vi "AutoAlign_N664_V2.vi"() -> ()   [LabVIEW 2014]
uses:
  Controls/StageStates.ctl
  Controls/GraphNotifier2D.ctl
panel:
  out "Current Step":i32
  in  "Done":bool
  in  "Repeat":bool
  in  "Start":bool
  out "Cursor Position":dbl=14.501547540983607
  in  "InitialStep":dbl=-0.5
  in  "StepSize":dbl=0.03
  in  "Number Of Steps":i32=35
  out "Intensity Graph":sgl[][](graph)=[[1575.0, 1530.0, 1467.0, 1650.0, 1682.0, 1613.0, 1536.0, 1626.0, 1940.0, 1831.0, 1587.0, 1388.0, 1511.0, 1435.0, 1379.0], [1709.0, 1679.0, 1771.0, 1769.0, 1775.0, 2008.0, 1804.0, 1975.0, 1770.0, 1847.0, 1595.0, 1554.0, 1478.0, 1427.0, 1513.0], [1648.0, 1736.0, 1646.0, 1749.0, 2076.0, 2140.0, 2064.0, 2285.0, 2553.0, 2003.0, 1778.0, 1592.0, 1374.0, 1409.0, 1484.0], [1691.0, 1662.0, 1787.0, 2129.0, 1967.0, 2135.0, 2802.0, 2654.0, 2620.0, 2152.0, 1653.0, 1625.0, 1294.0, 1626.0, 1484.0], [1791.0, 1866.0, 1955.0, 1940.0, 3130.0, 6076.0, 7812.0, 6999.0, 4445.0, 2270.0, 2108.0, 1656.0, 1663.0, 1432.0, 1434.0], [1685.0, 1692.0, 2032.0, 2360.0, 5595.0, 13786.0, 21952.0, 19970.0, 9456.0, 3969.0, 1980.0, 1953.0, 1670.0, 1777.0, 1482.0], [1690.0, 1883.0, 2231.0, 2992.0, 7277.0, 21162.0, 37225.0, 33877.0, 17031.0, 5558.0, 2486.0, 1757.0, 1705.0, 1721.0, 1629.0], [1950.0, 2070.0, 2444.0, 3114.0, 7300.0, 21633.0, 35295.0, 34230.0, 18542.0, 5857.0, 2447.0, 2046.0, 1718.0, 1496.0, 1497.0], [1738.0, 1911.0, 2271.0, 3013.0, 4517.0, 11402.0, 20736.0, 20231.0, 11390.0, 4490.0, 2670.0, 2143.0, 1981.0, 1468.0, 1542.0], [1875.0, 1741.0, 2051.0, 2522.0, 2677.0, 4632.0, 7218.0, 8580.0, 5418.0, 3381.0, 2550.0, 2068.0, 1621.0, 1690.0, 1591.0], [1727.0, 1602.0, 1790.0, 2337.0, 2453.0, 2325.0, 3198.0, 3570.0, 2998.0, 2777.0, 2034.0, 1844.0, 1659.0, 1637.0, 1530.0], [1562.0, 1616.0, 1920.0, 2051.0, 2025.0, 2333.0, 2346.0, 2577.0, 2301.0, 1999.0, 1878.0, 1700.0, 1628.0, 1624.0, 1486.0], [1599.0, 1666.0, 1677.0, 1735.0, 1646.0, 1710.0, 1950.0, 2008.0, 1755.0, 1922.0, 1644.0, 1723.0, 1616.0, 1341.0, 1659.0], [1496.0, 1555.0, 1749.0, 1781.0, 1666.0, 1880.0, 1703.0, 1865.0, 1750.0, 1712.0, 1685.0, 1646.0, 1592.0, 1380.0, 1439.0], [1706.0, 1543.0, 1659.0, 1490.0, 1552.0, 1610.0, 1653.0, 1799.0, 1670.0, 1665.0, 1578.0, 1393.0, 1625.0, 1681.0, 1501.0]]
  in  "Quit":bool
  out "Sample":cluster{dbl[], dbl[]}[](graph)
  in  "Accumulations":i32=10
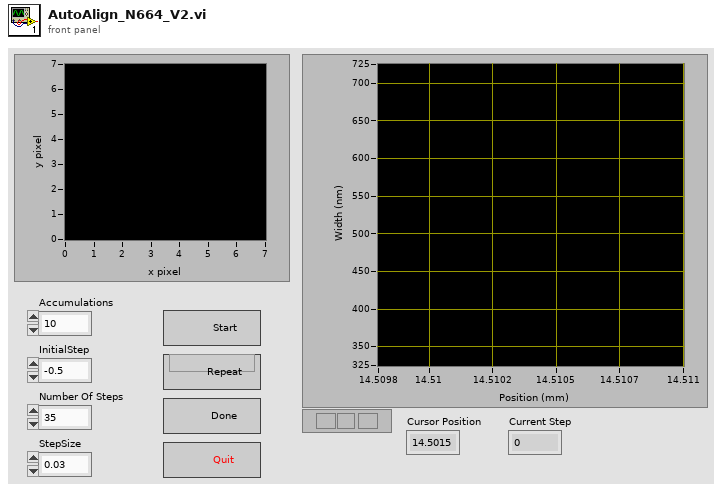
[diagram p1: front panel]
types:
  T1 = typedef "GraphNotifier2D.ctl" = cluster{"Xpos":i32, "Ypos":i32, "subarray":sgl[][], "Intensity":sgl}
  T2 = typedef "LabVIEW Interface for Arduino.lvlib/Arduino Resource.ctl" = cluster{"VISA resource":refnum<visa-resource-name>, "Board Type":T3, "Connection Type":enum8{"USB / Serial"}, "Bytes Per Packet (15)":u8}
  T3 = typedef "LabVIEW Interface for Arduino.lvlib/Board Type.ctl" = enum16{"Uno", "Dimuelanove w/Atmega 328", "Mega 2560"}
  T4 = typedef "StageStates.ctl" = enum16{"POSITION", "MVR", "MOVE", "HALT", "ONTARGET", "ERROR", "EXIT", "HOME", "ZEROPOS", "NANOPOS", "QUIT", "ANALOG"}
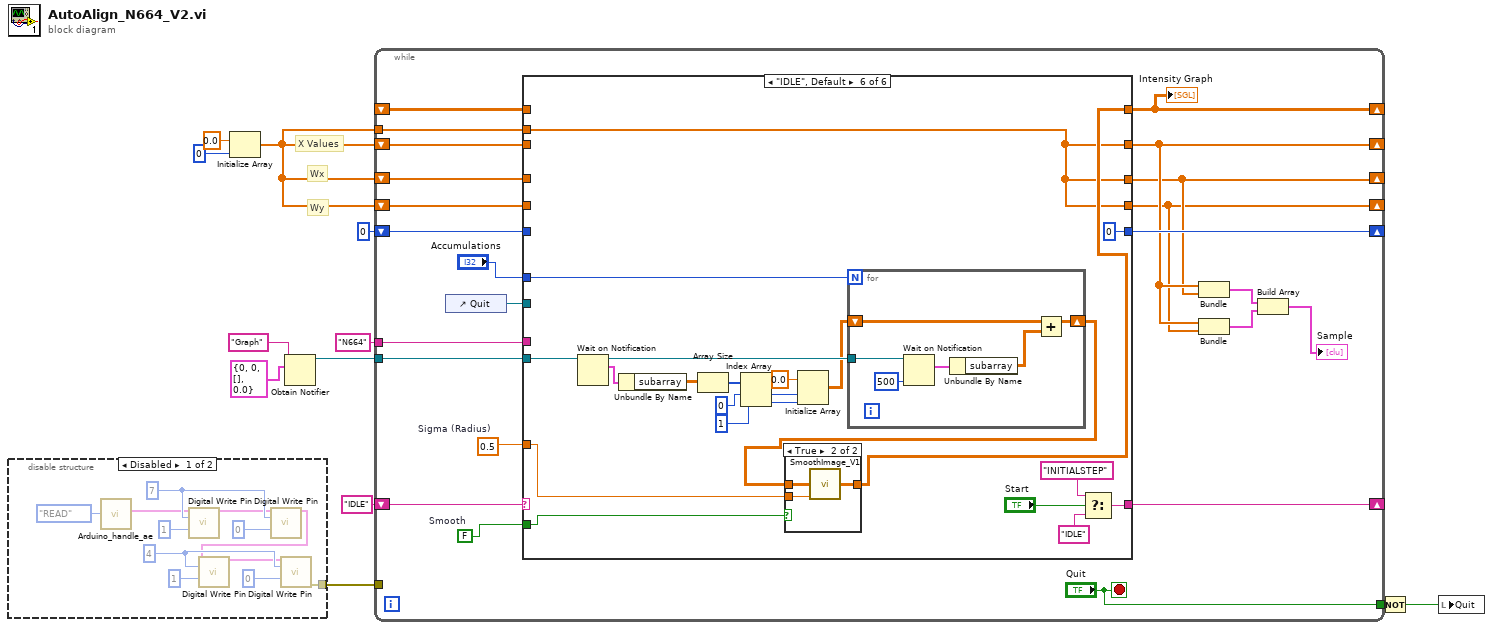
[diagram p0: block diagram]
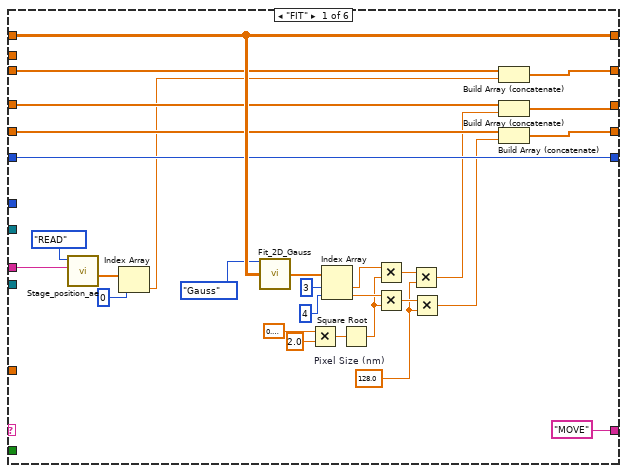
[diagram p3: hidden frame]
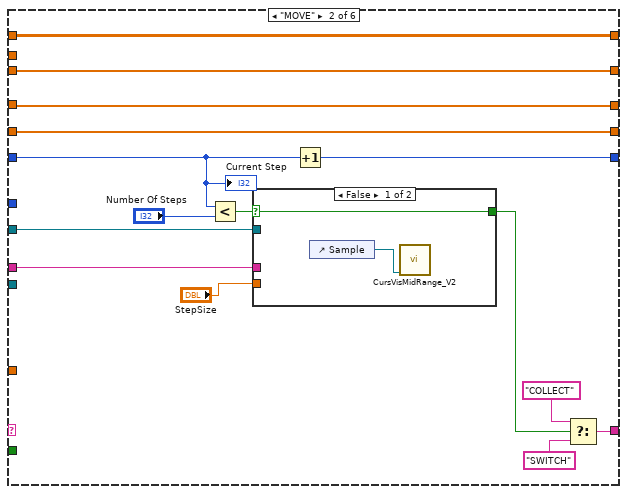
[diagram p4: hidden frame]
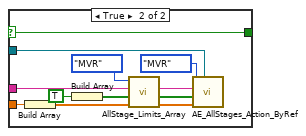
[diagram p5: hidden frame]
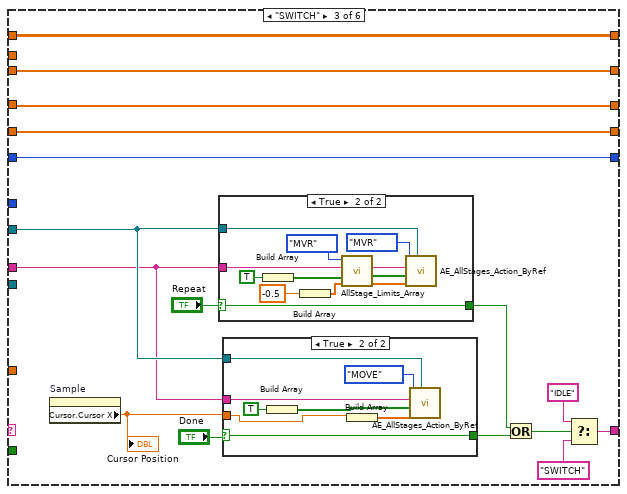
[diagram p6: hidden frame]
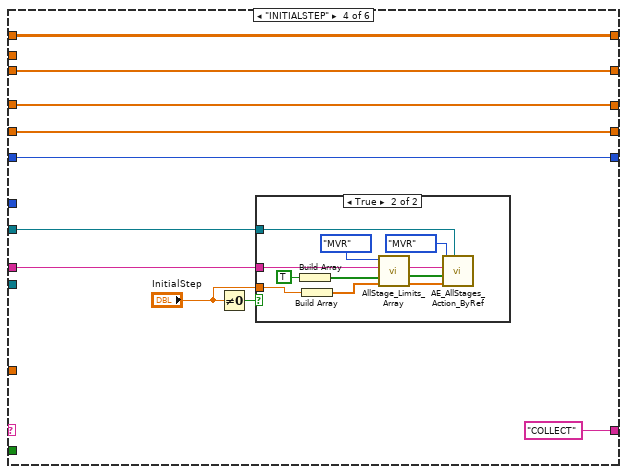
[diagram p9: hidden frame]
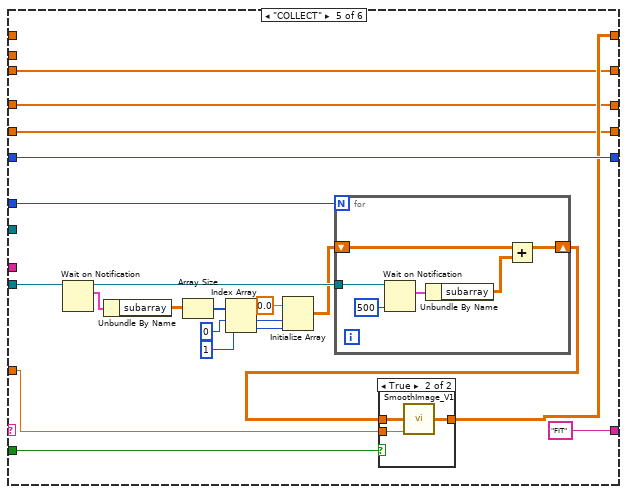
[diagram p11: hidden frame]
diagram:
  # "Wy"
  # "Wx"
  # "X Values"
  n1 = disable-structure shown="Disabled" {
    disable-tunnel: [w13 _] -> w9
    frame Disabled {
      w24 = u8 4 ("Digital I/O Pin (0)")
      w19 = u8 7 ("Digital I/O Pin (0)")
      n2 = call "Arduino_handle_ae.vi"("Enum"=enum16{"WRITE", "READ"}."READ") -> ("Arduino Resource Out"=w18:T2)  [unwired: 10 in]
      n3 = call <vilib>:"Digital Write Pin.vi"("Arduino Resource"=w18, "Digital I/O Pin (0)"=w19, "Value (0)"=u8 1) -> ("Arduino Resource"=w14:T2)  [unwired: 11 in, 1 out]
      n4 = call <vilib>:"Digital Write Pin.vi"("Arduino Resource"=w14, "Digital I/O Pin (0)"=w19, "Value (0)"=u8 0) -> ("Arduino Resource"=w23:T2)  [unwired: 11 in, 1 out]
      n5 = call <vilib>:"Digital Write Pin.vi"("Arduino Resource"=w23, "Digital I/O Pin (0)"=w24, "Value (0)"=u8 1) -> ("Arduino Resource"=w22:T2)  [unwired: 11 in, 1 out]
      n6 = call <vilib>:"Digital Write Pin.vi"("Arduino Resource"=w22, "Digital I/O Pin (0)"=w24, "Value (0)"=u8 0) -> ("error out"=w13:errorcluster)  [unwired: 11 in, 1 out]
    }
    frame Enabled {
    }
  }
  n7 = Initialize Array(0.0 ("element"), 0 ("dimension size")) -> (w1:dbl[])
  n8 = Obtain Notifier(name (unnamed)="Graph", notification data type=T1 {"Xpos"=0, "Ypos"=0, "subarray"=[], "Intensity"=0.0}) -> (notifier out=w6:refnum<notifier>)  [unwired: 2 in, 2 out]
  n9 = while {
    shift-right: [w46] -> _
    shift-left: _ -> [w47]
    shift-right: [w45] -> _
    shift-left: "IDLE" -> [w41]
    shift-right: [w43] -> _
    shift-left: 0 ("NumberOfSteps 2") -> [w44]
    tunnel: w6 -> [w40]
    tunnel: "N664" ("StageID") -> [w38]
    tunnel: w9 -> [_]
    tunnel: ["Quit"] -> w5
    tunnel: w1 -> [w25]
    shift-right: [w31] -> _
    shift-left: w1 -> [w34]
    shift-right: [w30] -> _
    shift-left: w1 -> [w33]
    shift-right: [w29] -> _
    shift-left: w1 -> [w32]
    stop <- "Quit" stop-if-true
    w36 = 0.5  # Sigma (Radius)
    w35 = FALSE  # Smooth
    n10 = control-ref of="Quit"() -> (w42:refnum<vi>)
    n11 = case shown="\"IDLE\", Default" w41 {
      tunnel: [w75 w91 w120 w153 w170 w197] -> w46
      tunnel: w47 -> [w75 w91 w120 w153 _ _]
      tunnel: w38 -> [w72 w82 w117 w149 _ _]
      tunnel: ["MOVE" w88 w114 "COLLECT" "FIT" w216] -> w45
      tunnel: w44 -> [w73 w86 w121 w152 w185 _]
      tunnel: [w73 w87 w121 w152 w185 0 ("NumberOfSteps 2")] -> w43
      tunnel: w42 -> [_ w84 w119 w151 _ _]
      tunnel: w40 -> [_ _ _ _ w174 w210]
      tunnel: "Accumulations" -> [_ _ _ _ w183 w213]
      tunnel: w36 -> [_ _ _ _ w169 w199]
      tunnel: w35 -> [_ _ _ _ w168 w200]
      tunnel: w34 -> [w57 w79 w108 w146 w167 _]
      tunnel: w33 -> [w56 w78 w107 w145 w166 _]
      tunnel: w32 -> [w55 w77 w106 w144 w165 _]
      tunnel: [w51 w79 w108 w146 w167 w196] -> w31
      tunnel: [w50 w78 w107 w145 w166 w196] -> w30
      tunnel: [w49 w77 w106 w144 w165 w196] -> w29
      tunnel: w25 -> [_ _ _ _ _ w196]
      frame "FIT" {
        w58 = 128.0  # Pixel Size (nm)
        n12 = call "Stage_position_ae.vi"("StageID"=w72, "Enum"=enum16{"WRITE", "READ"}."READ") -> ("Position Out"=w66:dbl[])  [unwired: 8 in, 1 out]
        n13 = Index Array(array=w66, index=0) -> (element=w54:dbl)
        n14 = call "Fit_2D_Gauss.vi"("Enum"=enum16{"Gauss", "Lorentz"}."Gauss", "Image IN"=w75) -> ("Fit Parameters"=w76:dbl[])  [unwired: 12 in, 1 out]
        n15 = Multiply(x=0.6931471805599453, y=2.0) -> (x*y=w69:dbl)
        n16 = Index Array(array=w76, index #1=3 ("index"), index #2=4 ("index")) -> (element #1=w68:dbl, element #2=w60:dbl)
        n17 = Square Root(x=w69) -> (sqrt(x)=w48:dbl)
        n18 = Multiply(x=w68, y=w48) -> (x*y=w61:dbl)
        n19 = Multiply(x=w60, y=w48) -> (x*y=w59:dbl)
        n20 = Multiply(x=w61, y=w58) -> (x*y=w53:dbl)
        n21 = Multiply(x=w59, y=w58) -> (x*y=w52:dbl)
        n22 = Build Array (concatenate)(w57, w54) -> (w51:dbl[])
        n23 = Build Array (concatenate)(w56, w53) -> (w50:dbl[])
        n24 = Build Array (concatenate)(w55, w52) -> (w49:dbl[])
      }
      frame "MOVE" {
        n25 = Less?(x=w86, y="Number Of Steps") -> (x < y?=w80:bool)
        n26 = case shown="False" w80 {
          selector: w80 -> [w93 w102]
          tunnel: w82 -> [_ w97]
          tunnel: w84 -> [_ w103]
          tunnel: [w93 w102] -> w85
          tunnel: "StepSize" -> [_ w95]
          frame False {
            n27 = control-ref of="Sample"() -> (w92:refnum<vi>)
            n28 = call "CursVisMidRange_V2.vi"("Sample 2"=w92) -> ()  [unwired: 11 in]
          }
          frame True {
            n29 = Build Array(w95) -> (w94:dbl[])
            n30 = Build Array(TRUE) -> (w98:bool[])
            n31 = call "AllStage_Limits_Array.vi"("Step(um)/Position(units)"=w94, "Axis"=w98, "Stage ID"=w97, "MOVE/MVR"=enum16{"MOVE", "MVR"}."MVR") -> ("Positions"=w99:dbl[], "Boolean Array"=w100:bool[], "Stage ID"=w101:string)  [unwired: 5 in]
            n32 = call "AE_AllStages_Action_ByRef.vi"("Abort"=w103, "Positions"=w99, "Axis"=w100, "Stage ID"=w101, "Action"=StageStates."MVR") -> ()  [unwired: 3 in, 4 out]
          }
        }
        n33 = Increment(x=w86) -> (x+1=w87:i32)
        n34 = Select(t="COLLECT", s=w85, f="SWITCH") -> (s? t:f=w88:string)
        "Current Step" <- w86
      }
      frame "SWITCH" {
        n35 = property on="Sample" class="XYGraph (strict)"() -> ("Cursor.Cursor X"=w118:dbl)  [unwired: 2 in, 2 out]
        "Cursor Position" <- w118
        n36 = case shown="True" "Repeat" {
          selector: "Repeat" -> [w131 w134]
          tunnel: w117 -> [_ w135]
          tunnel: w119 -> [_ w141]
          tunnel: [w131 w134] -> w110
          frame False {
          }
          frame True {
            n37 = Build Array(TRUE) -> (w140:bool[])
            n38 = Build Array(-0.5 ("Step(um)/Position(units)")) -> (w132:dbl[])
            n39 = call "AllStage_Limits_Array.vi"("Step(um)/Position(units)"=w132, "Axis"=w140, "Stage ID"=w135, "MOVE/MVR"=enum16{"MOVE", "MVR"}."MVR") -> ("Positions"=w137:dbl[], "Boolean Array"=w138:bool[], "Stage ID"=w139:string)  [unwired: 5 in]
            n40 = call "AE_AllStages_Action_ByRef.vi"("Abort"=w141, "Positions"=w137, "Axis"=w138, "Stage ID"=w139, "Action"=StageStates."MVR") -> ()  [unwired: 3 in, 4 out]
          }
        }
        n41 = case shown="True" "Done" {
          selector: "Done" -> [w122 w127]
          tunnel: w117 -> [_ w126]
          tunnel: w119 -> [_ w128]
          tunnel: w118 -> [_ w124]
          tunnel: [w122 w127] -> w109
          frame False {
          }
          frame True {
            n42 = Build Array(TRUE) -> (w125:bool[])
            n43 = Build Array(w124) -> (w123:dbl[])
            n44 = call "AE_AllStages_Action_ByRef.vi"("Abort"=w128, "Positions"=w123, "Axis"=w125, "Stage ID"=w126, "Action"=StageStates."MOVE") -> ()  [unwired: 3 in, 4 out]
          }
        }
        n45 = Or(x=w110, y=w109) -> (x .or. y?=w113:bool)
        n46 = Select(t="IDLE", s=w113, f="SWITCH") -> (s? t:f=w114:string)
      }
      frame "INITIALSTEP" {
        n47 = Not Equal To 0?(x="InitialStep") -> (x != 0?=w148:bool)
        n48 = case shown="True" w148 {
          tunnel: w149 -> [_ w160]
          tunnel: w151 -> [_ w162]
          tunnel: "InitialStep" -> [_ w161]
          frame False {
          }
          frame True {
            n49 = Build Array(TRUE) -> (w158:bool[])
            n50 = Build Array(w161) -> (w154:dbl[])
            n51 = call "AllStage_Limits_Array.vi"("Step(um)/Position(units)"=w154, "Axis"=w158, "Stage ID"=w160, "MOVE/MVR"=enum16{"MOVE", "MVR"}."MVR") -> ("Positions"=w155:dbl[], "Boolean Array"=w156:bool[], "Stage ID"=w157:string)  [unwired: 5 in]
            n52 = call "AE_AllStages_Action_ByRef.vi"("Abort"=w162, "Positions"=w155, "Axis"=w156, "Stage ID"=w157, "Action"=StageStates."MVR") -> ()  [unwired: 3 in, 4 out]
          }
        }
      }
      frame "COLLECT" {
        n53 = Wait on Notification(notifier=w174) -> (notifier out=w173:refnum<notifier>, notification=w182:T1)  [unwired: 3 in, 2 out]
        n54 = Unbundle By Name(w182) -> ("subarray"=w181:sgl[][])
        n55 = Array Size(array=w181) -> (size(s)=w180:i32[])
        n56 = Index Array(array=w180, index #1=0 ("index"), index #2=1 ("index")) -> (element #1=w177:i32, element #2=w176:i32)
        n57 = Initialize Array(sgl 0.0 ("element"), w177, w176) -> (w172:sgl[][])
        n58 = for {
          N: w183 -> [_]
          shift-right: [w195] -> w171
          shift-left: w172 -> [w194]
          tunnel: w173 -> [w192]
          n59 = Wait on Notification(notifier=w192, timeout in ms (-1)=500) -> (notification=w191:T1)  [unwired: 2 in, 3 out]
          n60 = Unbundle By Name(w191) -> ("subarray"=w190:sgl[][])
          n61 = Add(x=w194, y=w190) -> (x+y=w195:sgl[][])
        }
        n62 = case shown="True" w168 {
          tunnel: w171 -> [w186 w189]
          tunnel: [w186 w188] -> w170
          tunnel: w169 -> [_ w187]
          frame False {
          }
          frame True {
            n63 = call "SmoothImage_V1.vi"("Image IN"=w189, "Sigma (Radius)"=w187) -> ("Smoothed Image"=w188:sgl[][])  [unwired: 13 in]
          }
        }
      }
      frame "IDLE", Default {
        n64 = Wait on Notification(notifier=w210) -> (notifier out=w209:refnum<notifier>, notification=w212:T1)  [unwired: 3 in, 2 out]
        n65 = Unbundle By Name(w212) -> ("subarray"=w211:sgl[][])
        n66 = Array Size(array=w211) -> (size(s)=w208:i32[])
        n67 = Index Array(array=w208, index #1=0 ("index"), index #2=1 ("index")) -> (element #1=w205:i32, element #2=w204:i32)
        n68 = Initialize Array(sgl 0.0 ("element"), w205, w204) -> (w202:sgl[][])
        n69 = for {
          N: w213 -> [_]
          shift-right: [w227] -> w198
          shift-left: w202 -> [w226]
          tunnel: w209 -> [w224]
          n70 = Wait on Notification(notifier=w224, timeout in ms (-1)=500) -> (notification=w223:T1)  [unwired: 2 in, 3 out]
          n71 = Unbundle By Name(w223) -> ("subarray"=w222:sgl[][])
          n72 = Add(x=w226, y=w222) -> (x+y=w227:sgl[][])
        }
        n73 = case shown="True" w200 {
          tunnel: w198 -> [w218 w221]
          tunnel: [w218 w220] -> w197
          tunnel: w199 -> [_ w219]
          frame False {
          }
          frame True {
            n74 = call "SmoothImage_V1.vi"("Image IN"=w221, "Sigma (Radius)"=w219) -> ("Smoothed Image"=w220:sgl[][])  [unwired: 13 in]
          }
        }
        n75 = Select(t="INITIALSTEP", s="Start", f="IDLE") -> (s? t:f=w216:string)
      }
    }
    "Intensity Graph" <- w46
    n76 = Bundle(w31, w30) -> (w28:cluster{dbl[], dbl[]})  [unwired: 1 in]
    n77 = Bundle(w31, w29) -> (w27:cluster{dbl[], dbl[]})  [unwired: 1 in]
    n78 = Build Array(w28, w27) -> (→"Sample":cluster{dbl[], dbl[]}[])
  }
  n79 = Not(x=w5) -> (.not. x?=w4:bool)
  n80 = local write "Quit"(w4) -> ()
